vi "Check pos FM (SubVI).vi"(2 "error in":errorcluster, 3 "verify?":bool, 4 "VISA Refnum in":refnum<visa-resource-name>) -> (0 "error out":errorcluster, 1 "position":dbl)   [LabVIEW 2018]
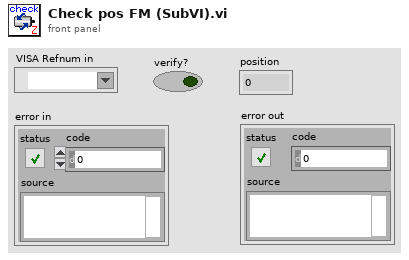
[diagram p1: front panel]
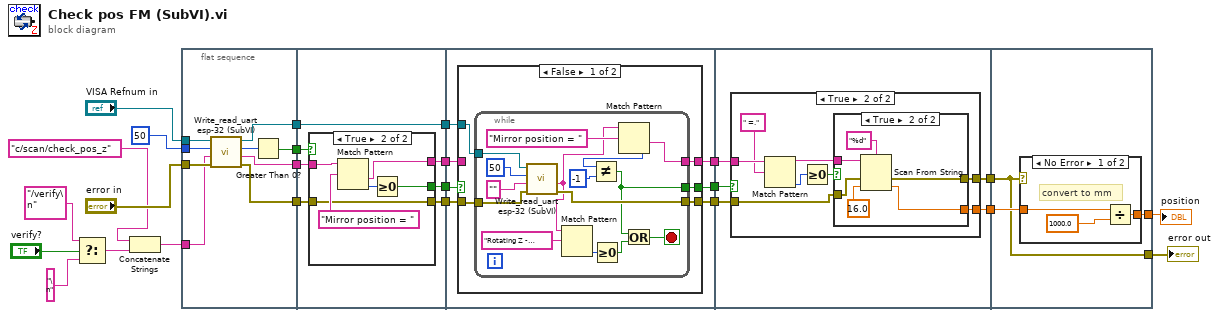
[diagram p0: block diagram]
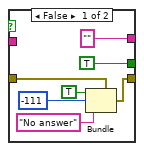
[diagram p2: hidden frame]
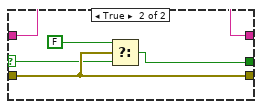
[diagram p3: hidden frame]
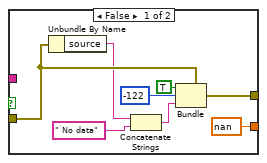
[diagram p4: hidden frame]
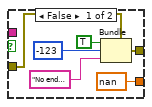
[diagram p5: hidden frame]
diagram:
  n1 = Select(t="/verify\n" ("string"), s="verify?", f="\n") -> (s? t:f=w2:string)
  n2 = Concatenate Strings("c/scan/check_pos_z" ("write buffer"), w2) -> (w1:string)
  n3 = flat-sequence {
    tunnel: u32 50 ("milliseconds to wait") -> [w33]
    tunnel: "error in" -> [w32]
    tunnel: "VISA Refnum in" -> [w31]
    tunnel: [w29] -> w21
    tunnel: [w28] -> w20
    tunnel: [w27] -> w19
    tunnel: [w26] -> w11
    tunnel: w1 -> [w25]
    tunnel: w21 -> [w40]
    tunnel: w20 -> [w39]
    tunnel: w19 -> [w38]
    tunnel: [w37] -> w18
    tunnel: [w36] -> w16
    tunnel: [w35] -> w14
    tunnel: [w34] -> w12
    tunnel: w11 -> [w34]
    tunnel: w18 -> [w60]
    tunnel: [w57] -> w17
    tunnel: w16 -> [w56]
    tunnel: [w55] -> w15
    tunnel: w14 -> [w59]
    tunnel: [w58] -> w13
    tunnel: w12 -> [w54]
    tunnel: w17 -> [w90]
    tunnel: w15 -> [w89]
    tunnel: w13 -> [w88]
    tunnel: [w87] -> w10
    tunnel: [w86] -> w9
    tunnel: w10 -> [w119]
    tunnel: w9 -> [w121]
    tunnel: [w120] -> w8
    tunnel: [w119] -> w7
    frame #0 {
      n4 = call "Write_read_uart esp-32 (SubVI).vi"("error in (no error)"=w32, "write buffer"=w25, "milliseconds to wait"=w33, "VISA Refnum in"=w31) -> ("error out 4"=w27:errorcluster, "read buffer"=w28:string, "read bite"=w30:u32, "VISA resource name out"=w26:refnum<visa-resource-name>)
      n5 = Greater Than 0?(x=w30) -> (x > 0?=w29:bool)
    }
    frame #1 {
      n6 = case shown="True" w40 {
        tunnel: w39 -> [_ w53]
        tunnel: w38 -> [w47 w48]
        tunnel: [TRUE w50] -> w37
        tunnel: ["" ("read buffer") w49] -> w36
        tunnel: [w43 w48] -> w35
        frame False {
          n7 = Bundle(cluster=w47, "status"=TRUE, "code"=-111, "source"="No answer") -> (w43:errorcluster)
        }
        frame True {
          n8 = Match Pattern(string=w53, regular expression="Mirror position = ") -> (after substring=w49:string, offset past match=w51:i32)  [unwired: 1 in, 2 out]
          n9 = Greater Or Equal To 0?(x=w51) -> (x >= 0?=w50:bool)
        }
      }
    }
    frame #2 {
      n10 = case shown="False" w60 {
        selector: w60 -> [_ w82]
        tunnel: w59 -> [w65 w85]
        tunnel: [w62 w85] -> w58
        tunnel: [w61 w83] -> w57
        tunnel: w56 -> [_ w84]
        tunnel: [w63 w84] -> w55
        tunnel: w54 -> [w64 _]
        frame False {
          n11 = while {
            tunnel: w65 -> [w78]
            tunnel: [w74] -> w62
            tunnel: [w72] -> w61
            tunnel: w64 -> [w67]
            tunnel: [w66] -> w63
            stop <- w75 stop-if-true
            n12 = call "Write_read_uart esp-32 (SubVI).vi"("error in (no error)"=w78, "write buffer"="", "milliseconds to wait"=u32 50, "VISA Refnum in"=w67) -> ("error out 4"=w74:errorcluster, "read buffer"=w68:string)  [unwired: 2 out]
            n13 = Match Pattern(string=w68, regular expression="Rotating Z - stopped!") -> (offset past match=w70:i32)  [unwired: 1 in, 3 out]
            n14 = Greater Or Equal To 0?(x=w70) -> (x >= 0?=w69:bool)
            n15 = Match Pattern(string=w68, regular expression="Mirror position = ") -> (after substring=w66:string, offset past match=w73:i32)  [unwired: 1 in, 2 out]
            n16 = Not Equal?(x=w73, y=-1 ("offset past match")) -> (x != y?=w72:bool)
            n17 = Or(x=w72, y=w69) -> (x .or. y?=w75:bool)
          }
        }
        frame True {
          n18 = Select(t=FALSE ("f"), s=w85, f=w82) -> (s? t:f=w83:bool)
        }
      }
    }
    frame #3 {
      n19 = case shown="True" w90 {
        tunnel: w89 -> [_ w106]
        tunnel: w88 -> [w94 w101]
        tunnel: [w96 w100] -> w87
        tunnel: [nan w99] -> w86
        frame False {
          n20 = Unbundle By Name(w94) -> ("source"=w92:string)
          n21 = Concatenate Strings(w92, " No data" ("source")) -> (w93:string)
          n22 = Bundle(cluster=w94, "status"=TRUE, "code"=-122, "source"=w93) -> (w96:errorcluster)
        }
        frame True {
          n23 = Match Pattern(string=w106, regular expression=" =.") -> (before substring=w102:string, offset past match=w104:i32)  [unwired: 1 in, 2 out]
          n24 = Greater Or Equal To 0?(x=w104) -> (x >= 0?=w103:bool)
          n25 = case shown="True" w103 {
            tunnel: w102 -> [_ w118]
            tunnel: w101 -> [w109 w115]
            tunnel: [w108 w114] -> w100
            tunnel: [nan w113] -> w99
            frame False {
              n26 = Bundle(cluster=w109, "status"=TRUE, "code"=-123, "source"="No end data") -> (w108:errorcluster)
            }
            frame True {
              n27 = Scan From String(format string="%d", input string=w118, error in=w115, default 1=16.0) -> (error out=w114:errorcluster, output 1=w113:dbl)  [unwired: 1 in, 2 out]
            }
          }
        }
      }
    }
    frame #4 {
      n28 = case shown="No Error" w119 {
        tunnel: w121 -> [w124 w125]
        tunnel: [w122 w125] -> w120
        frame No Error {
          # "convert to mm"
          n29 = Divide(x=w124, y=1000.0) -> (x/y=w122:dbl)
        }
        frame Error {
        }
      }
    }
  }
  "position" <- w8
  "error out" <- w7
